vi "CSGaussmeterGUI.contents.vi"   [LabVIEW 2014, in "CSGaussmeterGUI.lvlib"]
uses:
  CSGaussmeterGUI.lvlib
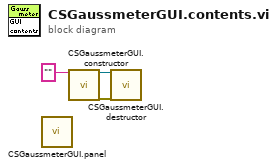
[diagram p0: block diagram]
diagram:
  n1 = call "CSGaussmeterGUI.panel.vi"() -> ()  [unwired: 1 in]
  n2 = call "CSGaussmeterGUI.constructor.vi"("name"="") -> ("i ref out"=w3:refnum<vi>, "error out"=w2:errorcluster)  [unwired: 16 in, 1 out]
  n3 = call "CSGaussmeterGUI.destructor.vi"("i ref in"=w3, "error in (no error)"=w2) -> ()  [unwired: 17 in, 1 out]
